vi "DIOToDash.vi"(7 "Name(DIO)":string="DIO", 8 "error in (no error)":errorcluster, 10 "Lead Screw Max":bool, 11 "Frisbee Catch":bool) -> (0 "error out":errorcluster)   [LabVIEW 2012]
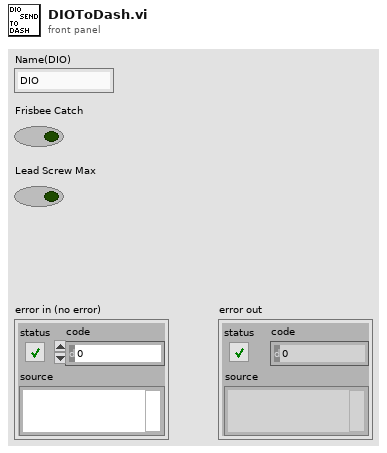
[diagram p1: front panel]
types:
  T1 = cluster{"Frisbee Catch":bool, "Lead Screw Max":bool}
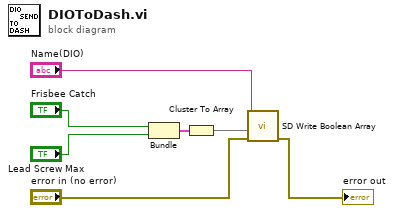
[diagram p0: block diagram]
diagram:
  n1 = Bundle("Frisbee Catch"="Frisbee Catch", "Lead Screw Max"="Lead Screw Max") -> (w4:T1)  [unwired: 1 in]
  n2 = Cluster To Array(cluster=w4) -> (array=w1:bool[])
  n3 = call <vilib>:"SD Write Boolean Array.vi"("error in"="error in (no error)", "Boolean Array"=w1, "Name"="Name(DIO)") -> ("error out"=→"error out":errorcluster)  [unwired: 7 in, 1 out]
